vi "NPC3SG Refresh v10.6.1.vi"(8 "error in":errorcluster caption="Fehler (Eingang - kein Fehler)", 9 "VISA-Ressourcen-Name (In)":refnum<visa-resource-name>, 11 "reset all":bool=TRUE) -> (3 "init ok??":bool)   [LabVIEW 2010]
uses:
  drivers/Newport NPC3SG/SubNPC3SG.llb/device variables.vi
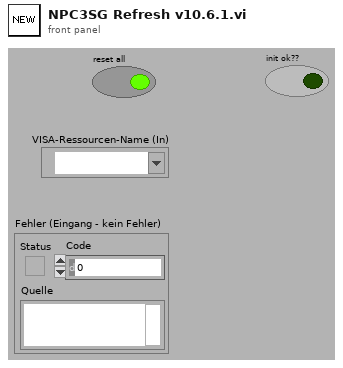
[diagram p1: front panel]
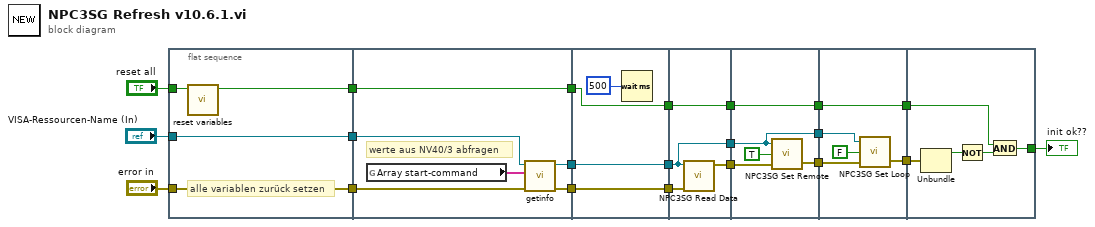
[diagram p0: block diagram]
diagram:
  n1 = flat-sequence {
    tunnel: "VISA-Ressourcen-Name (In)" -> [w23]
    tunnel: [w23] -> w17
    tunnel: "error in" -> [w22]
    tunnel: [w22] -> w16
    tunnel: "reset all" -> [w24]
    tunnel: [w25] -> w15
    tunnel: w17 -> [w30]
    tunnel: w16 -> [w29]
    tunnel: w15 -> [w28]
    tunnel: [w28] -> w11
    tunnel: [w27] -> w8
    tunnel: [w26] -> w7
    tunnel: w11 -> [w35]
    tunnel: [w35] -> w10
    tunnel: [w34] -> w9
    tunnel: w8 -> [w34]
    tunnel: w7 -> [w33]
    tunnel: [w33] -> w6
    tunnel: w10 -> [w39]
    tunnel: [w39] -> w12
    tunnel: w9 -> [w36]
    tunnel: w6 -> [w38]
    tunnel: [w37] -> w5
    tunnel: [w36] -> w4
    tunnel: w12 -> [w44]
    tunnel: [w44] -> w14
    tunnel: w5 -> [w42]
    tunnel: w4 -> [w40]
    tunnel: [w41] -> w3
    tunnel: [w40] -> w2
    tunnel: w14 -> [w49]
    tunnel: [w49] -> w13
    tunnel: w3 -> [w47]
    tunnel: w2 -> [w46]
    tunnel: [w45] -> w1
    tunnel: [w53] -> w19
    tunnel: w13 -> [w54]
    tunnel: w1 -> [w51]
    frame #0 {
      # "alle variablen zurück setzen"
      n2 = call "reset variables.vi"("reset all"=w24) -> ("init all ok"=w25:bool)  [unwired: 10 in]
    }
    frame #1 {
      # "werte aus NV40/3 abfragen"
      n3 = global read "device variables.vi" "Array start-command"() -> (w31:string[])
      n4 = call "getinfo.vi"("error in"=w29, "command array"=w31, "VISA-Ressourcen-Name (In)"=w30) -> ("error out"=w26:errorcluster, "VISA-Ressourcen-Name (Out)"=w27:refnum<visa-resource-name>)  [unwired: 7 in]
    }
    frame #2 {
      n5 = Wait (ms)(milliseconds to wait=u32 500 ("millisecond timer value")) -> ()  [unwired: 1 out]
    }
    frame #3 {
      n6 = call "NPC3SG Read Data.vi"("VISA resource name in"=w36, "error in"=w38) -> ("error ende"=w37:errorcluster)  [unwired: 8 in]
    }
    frame #4 {
      n7 = call "NPC3SG Set Remote.vi"("Get  Error"=w42, "Remote?"=TRUE, "Drive Visa Name"=w40) -> ("Send Error"=w41:errorcluster)  [unwired: 1 out]
    }
    frame #5 {
      n8 = call "NPC3SG Set Loop.vi"("Get  Error"=w47, "Close Loop?"=FALSE, "Drive Visa Name"=w46) -> ("Send Error"=w45:errorcluster)  [unwired: 1 out]
    }
    frame #6 {
      n9 = Unbundle(w51) -> ("status"=w52:bool)  [unwired: 2 out]
      n10 = Not(x=w52) -> (.not. x?=w50:bool)
      n11 = And(x=w54, y=w50) -> (x .and. y?=w53:bool)
    }
  }
  "init ok??" <- w19
